vi "FG_INI Data.vi"(8 "Error":errorcluster) -> (0 "Error Out":errorcluster, 3 "INI Data Out":T1 {"Body Text"."Body Text Spec"."Alignment" items=["left", "center", "right"]; "Text"."Alignment" items=["left", "center", "right"]}, 5 "Font List Out":string[](array[string]))   [LabVIEW 2021]
uses:
  TypeDefs/Cluster_INI Data.ctl
  vi.lib/LabVIEW Icon API/lv_icon/Controls/Font.ctl
  vi.lib/LabVIEW Icon API/lv_icon/Controls/Alignment.ctl
  TypeDefs/Num_Font Size.ctl
  TypeDefs/Cluster_BodyText.ctl
  vi.lib/LabVIEW Icon API/lv_icon/Controls/IEColor.ctl
  TypeDefs/Cluster_Button Draw Tools.ctl
  TypeDefs/Bool_Draw Tool.ctl
  TypeDefs/Bool_Line Tool.ctl
  TypeDefs/Bool_ColorExtractor Tool.ctl
  TypeDefs/Bool_Fill Tool.ctl
  TypeDefs/Bool_IERect Tool.ctl
  TypeDefs/Bool_FRect Tool.ctl
  TypeDefs/Bool_Circle Tool.ctl
  TypeDefs/Bool_FillCircle Tool.ctl
  TypeDefs/Bool_Eraser Tool.ctl
  TypeDefs/Bool_Text Tool.ctl
  TypeDefs/Bool_Selection Tool.ctl
  TypeDefs/Bool_Move Tool.ctl
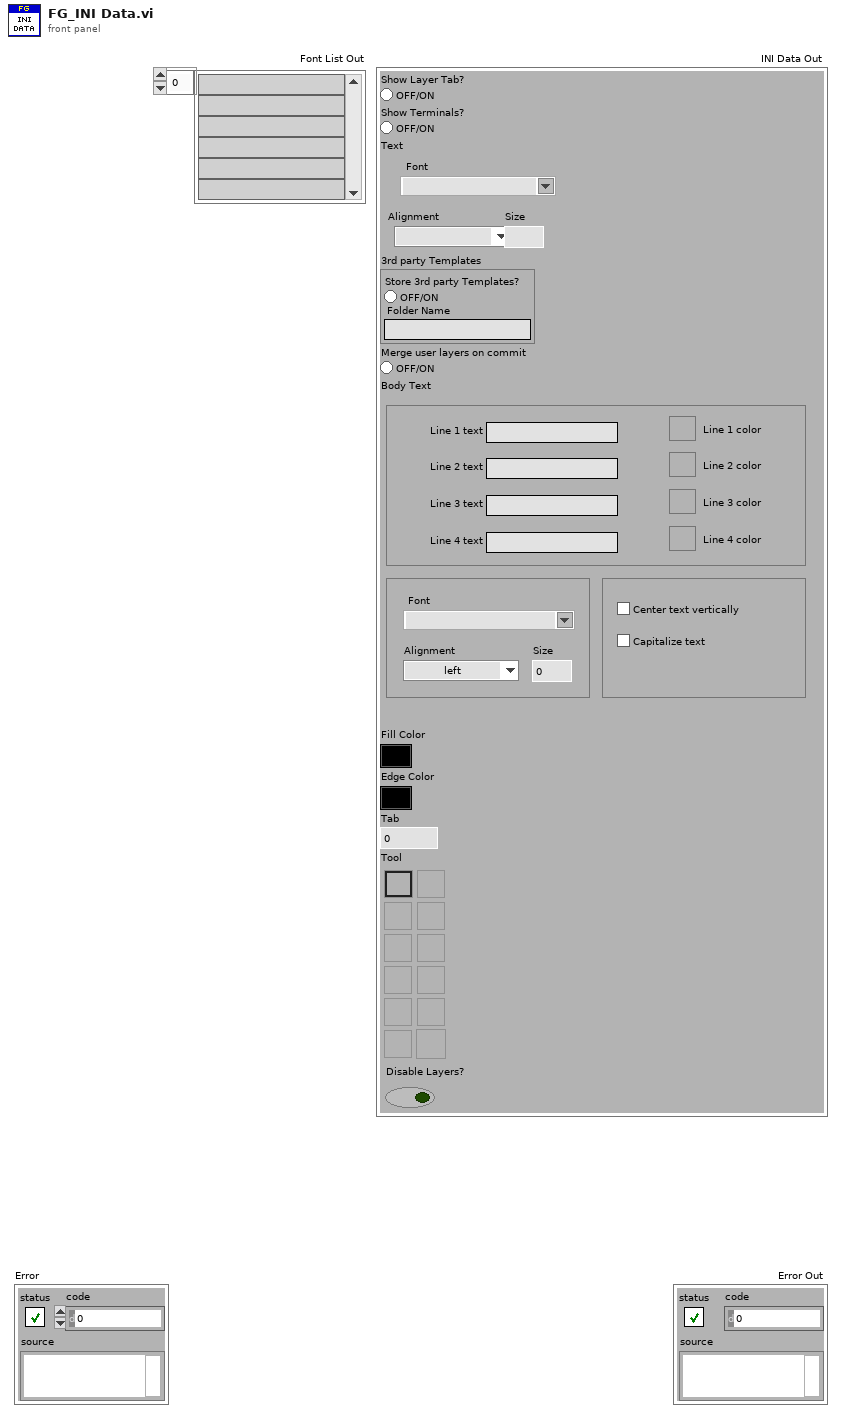
[diagram p1: front panel]
types:
  T1 = typedef "Cluster_INI Data.ctl" = cluster{"Show Layer Tab?":bool, "Show Terminals?":bool, "Text":cluster{"Font":T2, "Alignment":T3, "Size":T4}, "3rd party Templates":cluster{"Store 3rd party Templates?":bool, "Folder Name":string}, "Merge user layers on commit":bool, "Body Text":T5, "Fill Color":T6, "Edge Color":T6, "Tab":u16, "Tool":T7, "Disable Layers?":bool}
  T2 = typedef "Font.ctl" = string
  T3 = typedef "Alignment.ctl" = u16
  T4 = typedef "Num_Font Size.ctl" = u8
  T5 = typedef "Cluster_BodyText.ctl" = cluster{"Line 1 text":string, "Line 2 text":string, "Line 3 text":string, "Line 4 text":string, "Line 1 color":u32, "Line 2 color":u32, "Line 3 color":u32, "Line 4 color":u32, "Body Text Spec":cluster{"Font":T2, "Alignment":T3, "Size":u8}, "Center text vertically":bool, "Capitalize Text":bool}
  T6 = typedef "IEColor.ctl" = u32
  T7 = typedef "Cluster_Button Draw Tools.ctl" = enum32{"Pencil", "Line", "Dropper", "Fill", "Rectangle", "Filled Rectangle", "Ellipse", "Filled Ellipse", "Eraser", "Text", "Select", "Move"}
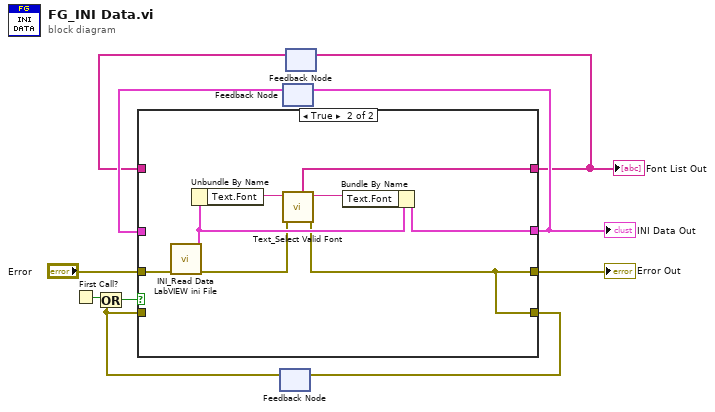
[diagram p0: block diagram]
diagram:
  n1 = First Call?() -> (First Call?: T/F=w10:bool)
  n2 = feedback #1() -> (w5:errorcluster)  [unwired: 1 in]
  n3 = Or(x=w10, y=w5) -> (x .or. y?=w6:bool)
  n4 = feedback #2() -> (w8:T1)  [unwired: 1 in]
  n5 = feedback #3() -> (w1:string[])  [unwired: 1 in]
  n6 = case shown="True" w6 {
    tunnel: [w14 w15] -> w4
    tunnel: [w13 w18] -> w7
    tunnel: "Error" -> [w14 w22]
    tunnel: w8 -> [w13 _]
    tunnel: w5 -> [w12 _]
    tunnel: [w12 w15] -> w3
    tunnel: [w11 w20] -> w2
    tunnel: w1 -> [w11 _]
    frame False {
    }
    frame True {
      n7 = call "INI_Read Data LabVIEW ini File.vi"("Error"=w22) -> ("Error Out"=w16:errorcluster, "INI Data Out"=w19:T1)  [unwired: 1 in, 8 out]
      n8 = Unbundle By Name(w19) -> ("Text.Font"=w21:T2)
      n9 = call "Text_Select Valid Font.vi"("Error"=w16, "Font"=w21) -> ("Error Out"=w15:errorcluster, "Valid Font Name Out"=w17:string, "Font List Out"=w20:string[])  [unwired: 7 in]
      n10 = Bundle By Name(cluster=w19, "Text.Font"=w17) -> (w18:T1)
    }
  }
  "INI Data Out" <- w7
  "Error Out" <- w4
  "Font List Out" <- w2
  n11 = feedback-in #1(w3) -> ()
  n12 = feedback-in #2(w7) -> ()
  n13 = feedback-in #3(w2) -> ()
